vi "Get Transfer Buffers.vi"(7 "transfer id":i32, 8 "error in (no error)":errorcluster, 9 "group id":i32, 10 "plugin id":i32, 11 "Buffers Map in":refnum<class "Buffers Map.lvclass">) -> (0 "error out":errorcluster, 1 "string Buffer":refnum<class "Buffer.lvclass">, 2 "engine Buffer":refnum<class "Buffer.lvclass">, 3 "Buffers Map out":refnum<class "Buffers Map.lvclass">)   [LabVIEW 2017, in "DSF Core.lvlib" / "Buffers Map.lvclass"]
uses:
  Buffers Map.lvclass
  Buffer/Buffer.lvclass
  Buffers Map.lvclass/Buffers Map.ctl
  Transfer/Transfer.lvclass
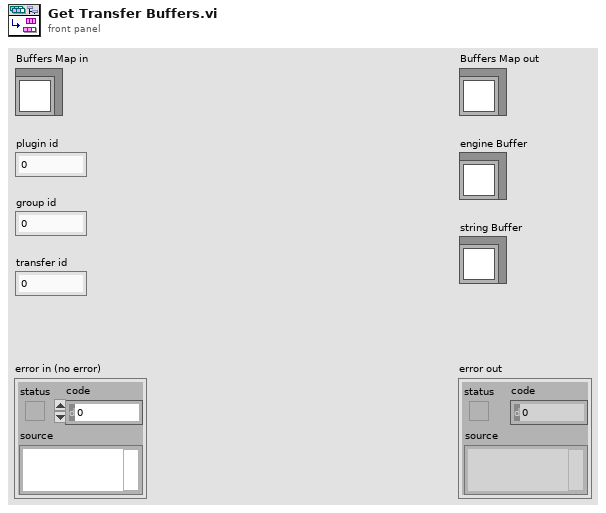
[diagram p1: front panel]
types:
  T1 = typedef "DSF Core.lvlib/Buffers Map.lvclass/Plugin.ctl" = cluster{"Plugin Buffers":refnum<class "Buffers.lvclass">, "Groups":T2[]}
  T2 = typedef "DSF Core.lvlib/Buffers Map.lvclass/Group.ctl" = cluster{"Group Buffers":refnum<class "Buffers.lvclass">, "Transfers":refnum<class "Transfer.lvclass">[]}
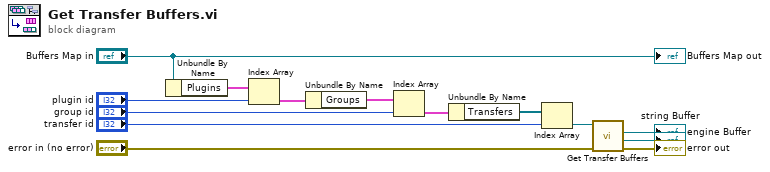
[diagram p0: block diagram]
diagram:
  n1 = Unbundle By Name("Buffers Map in") -> ("Plugins"=w13:T1[])
  n2 = Index Array(array=w13, index="plugin id") -> (element=w11:T1)
  n3 = Unbundle By Name(w11) -> ("Groups"=w10:T2[])
  n4 = Index Array(array=w10, index="group id") -> (element=w8:T2)
  n5 = Unbundle By Name(w8) -> ("Transfers"=w7:refnum<class "Transfer.lvclass">[])
  n6 = Index Array(array=w7, index="transfer id") -> (element=w5:refnum<class "Transfer.lvclass">)
  n7 = call "Get Transfer Buffers.vi"("error in (no error)"="error in (no error)", "Transfer in"=w5) -> ("error out"=→"error out":errorcluster, "string Buffer"=→"string Buffer":refnum<class "Buffer.lvclass">, "engine Buffer"=→"engine Buffer":refnum<class "Buffer.lvclass">)  [unwired: 6 in, 1 out]
  "Buffers Map out" <- "Buffers Map in"
